vi "Ethernet_connection_test_VISA.vi"() -> ()   [LabVIEW 2017]
uses:
  <vilib>/Utility/error.llb/DialogType.ctl
panel:
  in  "error in (no error)":errorcluster
  out "error out":errorcluster
  in  "VISA resource name":refnum<visa-resource-name>="AKIP"
  out "read buffer":string
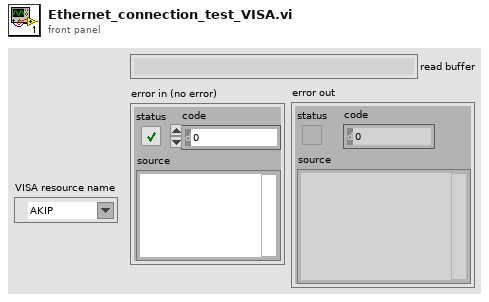
[diagram p1: front panel]
types:
  T1 = typedef "DialogType.ctl" = u16
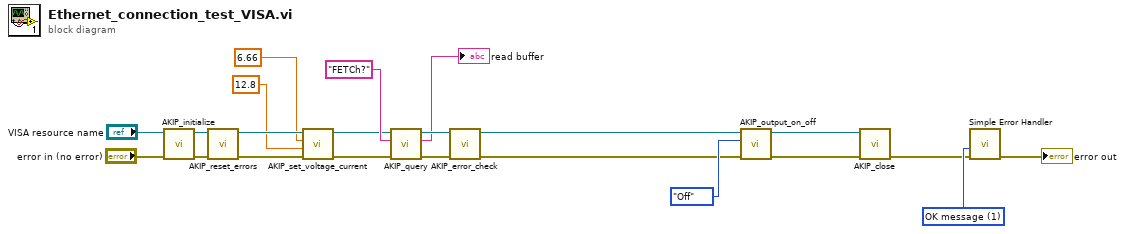
[diagram p0: block diagram]
diagram:
  w22 = T1 1 items=["no dialog", "OK message", "continue or stop message", "OK message + warnings", "continue/stop + warnings"] ("type of dialog (OK msg:1)")
  n1 = call "AKIP_initialize.vi"("error in (no error)"="error in (no error)", "VISA Refnum in"="VISA resource name") -> ("error out"=w14:errorcluster, "VISA Refnum out"=w13:refnum<visa-resource-name>)  [unwired: 8 in]
  n2 = call "AKIP_reset_errors.vi"("error in (no error)"=w14, "VISA Refnum in"=w13) -> ("error out"=w3:errorcluster, "VISA Refnum out"=w6:refnum<visa-resource-name>)  [unwired: 8 in]
  n3 = call "AKIP_set_voltage_current.vi"("error in (no error)"=w3, "Current"=12.8 ("value (0)"), "Voltage"=6.66 ("value (0)"), "VISA resource name (in)"=w6) -> ("error out"=w4:errorcluster, "VISA resource name (out)"=w5:refnum<visa-resource-name>)  [unwired: 6 in]
  n4 = call "AKIP_query.vi"("error in (no error)"=w4, "write buffer"="FETCh?", "VISA Refnum in"=w5) -> ("error out"=w16:errorcluster, "read buffer"=→"read buffer":string, "VISA Refnum out"=w15:refnum<visa-resource-name>)  [unwired: 6 in]
  n5 = call "AKIP_error_check.vi"("error in (no error)"=w16, "VISA Refnum in"=w15) -> ("error out"=w8:errorcluster, "VISA Refnum out"=w9:refnum<visa-resource-name>)  [unwired: 8 in]
  n6 = call "AKIP_output_on_off.vi"("error in (no error)"=w8, "Enum"=enum16{"On", "Off"}."Off", "VISA Refnum in"=w9) -> ("error out"=w11:errorcluster, "VISA Refnum out"=w12:refnum<visa-resource-name>)  [unwired: 7 in]
  n7 = call "AKIP_close.vi"("error in (no error)"=w11, "VISA Refnum in"=w12) -> ("error out"=w21:errorcluster)  [unwired: 8 in, 1 out]
  n8 = call <vilib>:"Simple Error Handler.vi"("type of dialog (OK msg:1)"=w22, "error in (no error)"=w21) -> ("error out"=→"error out":errorcluster)  [unwired: 3 in, 4 out]
